vi "Wrapper_Create_Mod.vi"(8 "error in (no error)":errorcluster caption="entrée d'erreur (pas d'erreur)") -> (0 "error out":errorcluster caption="sortie d'erreur", 1 "Wrapper":u32)   [LabVIEW 2024]
uses:
  Program Files (x86)/Ocean Optics/OmniDriver/OOI_HOME/OmniDriver32.dll
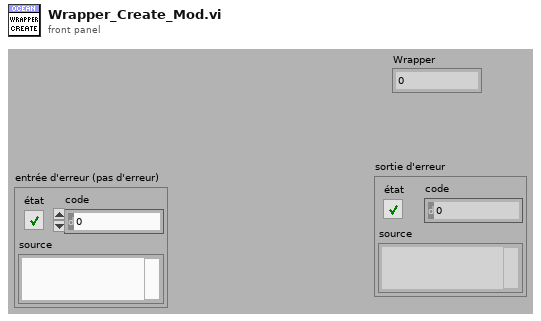
[diagram p1: front panel]
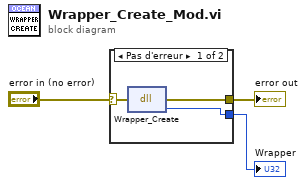
[diagram p0: block diagram]
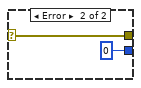
[diagram p2: hidden frame]
diagram:
  n1 = case shown="Pas d'erreur" "error in (no error)" {
    selector: "error in (no error)" -> [w5 w7]
    tunnel: [w6 u32 0] -> w3
    tunnel: [w4 w7] -> w1
    frame No Error {
      n2 = dll-call lib="C:/Program Files (x86)/Ocean Optics/OmniDriver/OOI_HOME/OmniDriver32.dll" fn="Wrapper_Create" label="Wrapper.Create"(error in=w5) -> (error out=w4:errorcluster, "type de retour"=w6:u32)  [unwired: 2 in, 1 out]
    }
    frame Error {
    }
  }
  "Wrapper" <- w3
  "error out" <- w1
